vi "Linear Sweep.vi"(0 "Start":dbl=1.0, 5 "End":dbl=1.0, 7 "Delta":dbl format="%#_13g", 11 "error in (no error)":errorcluster) -> (4 "Ramp Pattern":dbl[](array[numeric]), 15 "error out":errorcluster)   [LabVIEW 2020]
doc: "Linear Sweep performs a linear sweep from start to stop in steps of delta value passed as an input."
uses:
  <vilib>/Analysis/1siggen.llb/Ramp Pattern by Delta.vi
  <vilib>/Analysis/NI_AALBase.lvlib
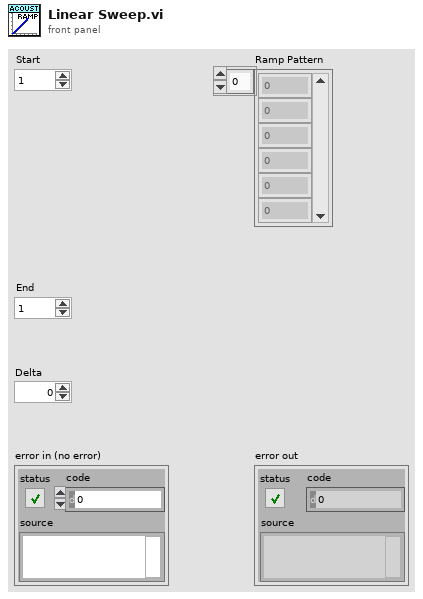
[diagram p1: front panel]
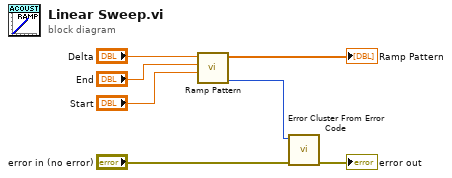
[diagram p0: block diagram]
diagram:
  n1 = call-poly <vilib>:"Ramp Pattern.vi"("start"="Start", "end"="End", "delta"="Delta") -> ("error"=w4:i32, "Ramp Pattern"=→"Ramp Pattern":dbl[])  [unwired: 6 in, 1 out]
  n2 = call <vilib>:"Error Cluster From Error Code.vi"("error in (no error)"="error in (no error)", "error code (0)"=w4) -> ("error out"=→"error out":errorcluster)  [unwired: 7 in]
